vi "Define.vi"() -> (3 "ID out":refnum<class "ID.lvclass">)   [LabVIEW 2022 SP3, in "Conditum.lvlib" / "Columns.lvlib" / "ID.lvclass"]
uses:
  ID.lvclass
  ID.lvclass/ID.ctl
  Type/Type.lvclass
  Type/Definition.ctl
  Attributes.ctl
  Conditum.lvlib
  LabVIEW Type.ctl
  C:/dev/lv/illuminated-g/lv-conditum/Conditum/Columns/Type/Type.lvclass
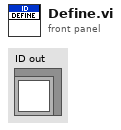
[diagram p1: front panel]
types:
  T1 = typedef "Conditum.lvlib/LabVIEW Type.ctl" = enum16{"None", "ID", "Boolean", "Integer", "Double", "Timestamp", "String", "Text", "Entity"}
  T2 = typedef "Conditum.lvlib/Attributes.ctl" = cluster{"Primary Key":bool, "Unique":bool, "Foreign Key":bool, "Auto Increment":bool}
  T3 = typedef "Conditum.lvlib/Columns.lvlib/Type.lvclass/Definition.ctl" = cluster{"Name":string, "Nullable":bool, "Default NULL":bool}
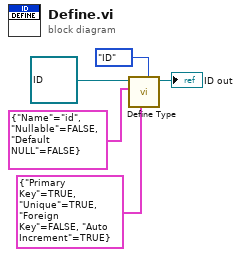
[diagram p0: block diagram]
diagram:
  n1 = call "Define Type.vi"("Type"=LabVIEW_Type."ID", "Attributes"=T2 {"Primary Key"=TRUE, "Unique"=TRUE, "Foreign Key"=FALSE, "Auto Increment"=TRUE}, "Definition"=T3 {"Name"="id", "Nullable"=FALSE, "Default NULL"=FALSE}, "Type in"=refnum<class "ID.lvclass"> refnum ("ID out")) -> ("Type out"=→"ID out":refnum<class "ID.lvclass">)  [unwired: 7 in]
